vi "HomeMotors.vi"(8 "error in (no error)":errorcluster, 11 "MotorController in":refnum<class "MotorController.lvclass">) -> (0 "error out":errorcluster, 3 "MotorController out":refnum<class "MotorController.lvclass">)   [LabVIEW 2019, in "MotorController.lvclass"]
uses:
  MotorController.lvclass
  MotorController.lvclass/MotorController.ctl
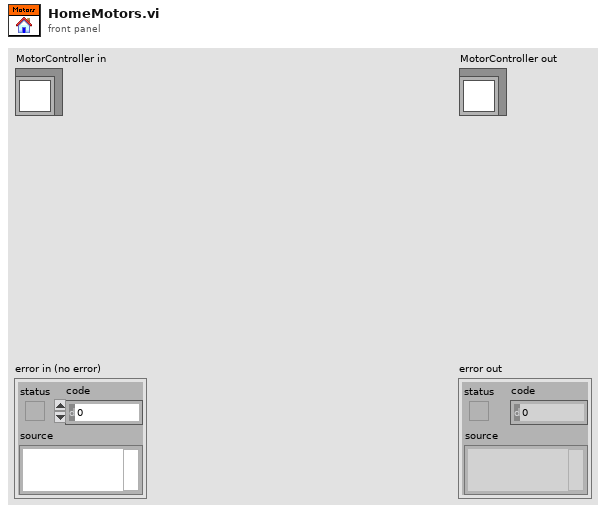
[diagram p1: front panel]
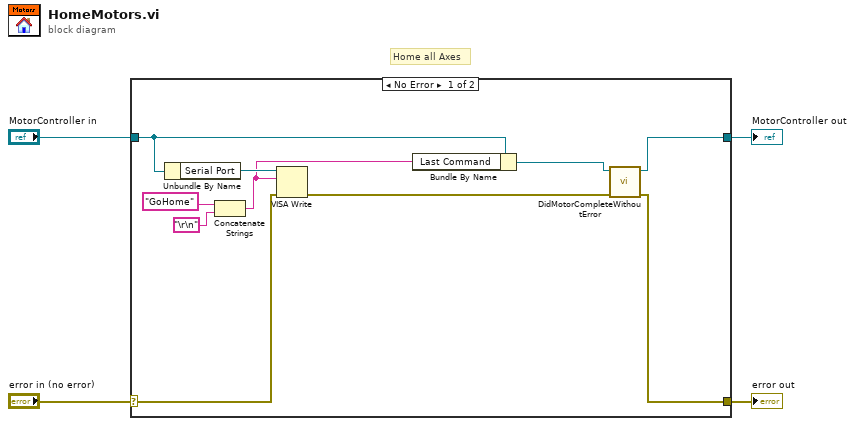
[diagram p0: block diagram]
diagram:
  # "Home all Axes"
  n1 = case shown="No Error" "error in (no error)" {
    selector: "error in (no error)" -> [w11 w16]
    tunnel: [w8 w16] -> w3
    tunnel: [w10 w15] -> w1
    tunnel: "MotorController in" -> [w7 w15]
    frame No Error {
      n2 = Unbundle By Name(w7) -> ("Serial Port"=w14:refnum<visa-resource-name>)
      n3 = Concatenate Strings("GoHome", "\r\n") -> (w5:string)
      n4 = VISA Write(VISA resource name=w14, write buffer=w5, error in (no error)=w11) -> (error out=w9:errorcluster)  [unwired: 2 out]
      n5 = Bundle By Name(cluster=w7, "Last Command"=w5) -> (w6:refnum<class "MotorController.lvclass">)
      n6 = call "DidMotorCompleteWithoutError.vi"("error in (no error)"=w9, "MotorController in"=w6) -> ("error out"=w8:errorcluster, "MotorController out"=w10:refnum<class "MotorController.lvclass">)  [unwired: 7 in, 1 out]
    }
    frame Error {
    }
  }
  "error out" <- w3
  "MotorController out" <- w1
